vi "Untitled 8.vi"   [LabVIEW 2017]
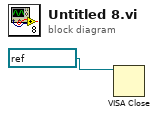
[diagram p0: block diagram]
diagram:
  n1 = VISA Close(VISA resource name=refnum<visa-resource-name> "COM13") -> ()  [unwired: 1 in, 1 out]
